vi "Launch Daemon.vi"(11 "MenuButton Event Handler in":refnum<class "MenuButton Event Handler.lvclass">) -> (0 "error out":errorcluster, 3 "MenuButton Event Handler out":refnum<class "MenuButton Event Handler.lvclass">)   [LabVIEW 2017, in "MenuButtons.lvlib" / "MenuButton Event Handler.lvclass"]
uses:
  MenuButton Event Handler.lvclass
  Daemon.vi
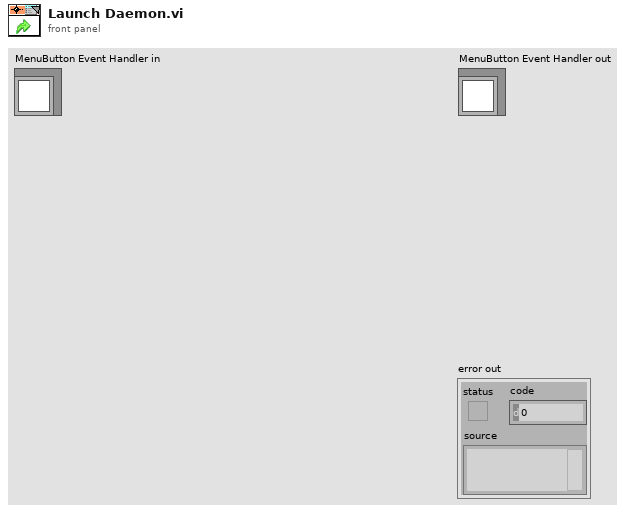
[diagram p1: front panel]
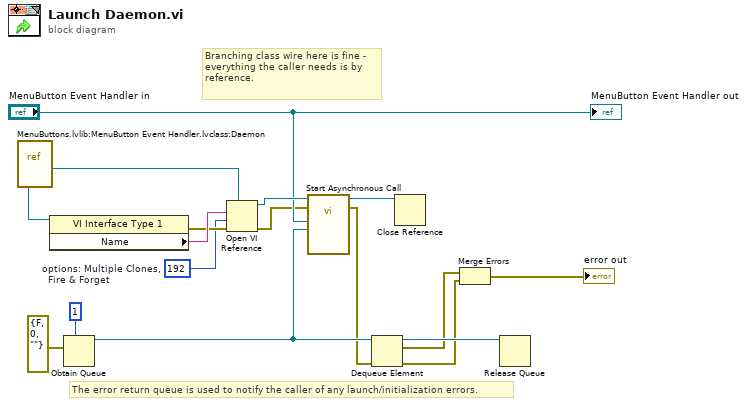
[diagram p0: block diagram]
diagram:
  w13 = 192  # options: Multiple Clones,   Fire & Forget
  # "Branching class wire here is fine - everything the caller needs is by reference."
  # "The error return queue is used to notify the caller of any launch/initialization errors."
  n1 = vi-ref "MenuButtons.lvlib:MenuButton Event Handler.lvclass:Daemon.vi"() -> (w16:refnum<vi>)
  n2 = property class="VI Interface Type 1"(reference=w16) -> (error out=w14:errorcluster, "Name"=w15:string)  [unwired: 1 in, 1 out]
  n3 = Obtain Queue(max queue size (-1, unlimited)=1, element data type=errorcluster {"status"=FALSE, "code"=0, "source"=""} ("error in (no error)")) -> (queue out=w7:refnum<queue>)  [unwired: 3 in, 2 out]
  n4 = Open VI Reference(type specifier VI Refnum (for type only)=w16, vi path=w15, options=w13, error in (no error)=w14) -> (vi reference=w12:refnum<vi>, error out=w8:errorcluster)  [unwired: 2 in]
  n5 = call-by-ref "Start Asynchronous Call"(reference=w12, error in=w8, "Return Queue"=w7, "MenuButton Event Handler in"="MenuButton Event Handler in") -> (reference out=w1:refnum<vi>, error out=w6:errorcluster)  [unwired: 10 in]
  n6 = Dequeue Element(queue=w7, error in (no error)=w6) -> (queue out=w5:refnum<queue>, element=w4:errorcluster, error out=w2:errorcluster)  [unwired: 1 in, 1 out]
  n7 = Close Reference(reference=w1) -> ()  [unwired: 1 in, 1 out]
  n8 = Merge Errors(w4, w2) -> (→"error out":errorcluster)
  n9 = Release Queue(queue=w5) -> ()  [unwired: 2 in, 3 out]
  "MenuButton Event Handler out" <- "MenuButton Event Handler in"
